vi "NI5112.destructor.vi"(0 "i ref in":refnum<vi>, 5 "error in(no error)":errorcluster) -> (19 "error out":errorcluster)   [LabVIEW 2014, in "NI5112.lvlib"]
doc: "This is the destructor of a class.\n\nLicense Agreement for this software:\n\nCopyright (C)\nGesellschaft für Schwerionenforschung, GSI\nPlanckstr. 1\n64291 Darmstadt\nGermany\n\nContact: D.Beck@gsi.de \n\nThis program is free software; you can redistribute it and/or modify it under the terms of the \nGNU General Public License as published by the Free Software Foundation; either version 2 of \nthe license, or (at your option) any later version.\n\nThis program is distributed in the hope that it will be useful, but WITHOUT ANY WARRANTY; \nwithout even the implied warranty of MERCHANTABILITY or FITNESS FOR A PARTICULAR PURPOSE. See the GNU General License for more details (http://www.gnu.org).\n\nGesellschaft für Schwerionenforschung, GSI\nPlanckstr. 1, 64291 Darmstadt, Germany\nFor all questions and ideas contact: M.Richter@gsi.de, H.Brand@gsi.de or D.Beck@gsi.de.\nLast update: 16-JUN-2004"
uses:
  NI5112.lvlib
  CSCore/BaseProcess/BaseProcess.lvlib
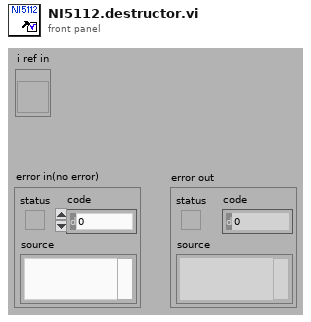
[diagram p1: front panel]
types:
  T1 = enum16{"SetAttribute", "GetAttribute", "CreateAttribute", "DestroyAttribute", "DestroyAllAtributes"}
  T2 = typedef "NI5112.lvlib/NI5112.i attribute.ctl" = cluster{"HWChannel":string, "instrument handle":refnum<k15>, "BinWidth":dbl, "vertical offset":dbl, "vertical range":dbl, "DataBPR":i32, "5112BPR":i32, "FullSpeed":bool, "discrLevel":dbl, "DoDiscr":bool, "VerCoupling":string}
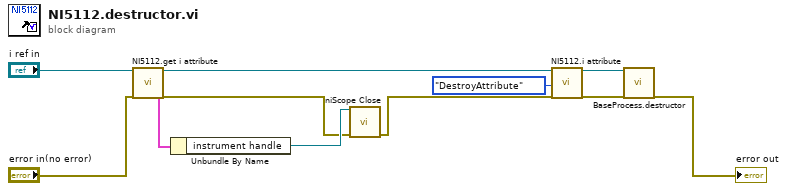
[diagram p0: block diagram]
diagram:
  n1 = call "NI5112.get i attribute.vi"("i ref in"="i ref in", "error in (no error)"="error in(no error)") -> ("i ref out"=w5:refnum<vi>, "i attribute"=w4:T2, "error out"=w2:errorcluster)  [unwired: 15 in]
  n2 = Unbundle By Name(w4) -> ("instrument handle"=w3:refnum<k15>)
  n3 = call <instrlib>:"niScope Close.vi"("instrument handle"=w3, "error in"=w2) -> ("error out"=w1:errorcluster)  [unwired: 13 in]
  n4 = call "NI5112.i attribute.vi"("VI Refnum"=w5, "Action"=T1."DestroyAttribute", "error in (no error)"=w1) -> ("VI Refnum out"=w10:refnum<vi>, "error out"=w9:errorcluster)  [unwired: 14 in, 1 out]
  n5 = call "BaseProcess.destructor.vi"("i ref in"=w10, "error in (no error)"=w9) -> ("error out"=→"error out":errorcluster)  [unwired: 17 in]
